vi "MSGR Receive (Name).vi"(0 "MSGR Q name":T2, 11 "error in (no error)":errorcluster, 12 "timeout in ms (-1)":i32=-1) -> (6 "MSGR Q Data TypeDef":T1, 14 "timed out?":bool, 15 "error out":errorcluster)   [LabVIEW 2018]
doc: "$Author::Richard Jennings $\n$Rev:: $\n$Date:: May, 2008 $\n\nOVERVIEW:\nReentrant VI to receive messages via a MSGR Q. If the Q does not exist this VI will create it, then wait for data.\n\nINPUTS (Controls):\n<name> - <short description of each control wired to connector pane>\n\nOUTPUTS (Indicators):\n<name> - <short description of each indicator wired to connector pane>\n\nCopyright 2008 - 2016 Jennings Embedded Servies. All rights reserved.\nAuthor makes no warranties or guarantees related to performance of the software.\nUSE AT YOUR OWN RISK\nwww.jembedded.com"
uses:
  MSGR Q Name TypeDef.ctl
  MSGR Q Data TypeDef.ctl
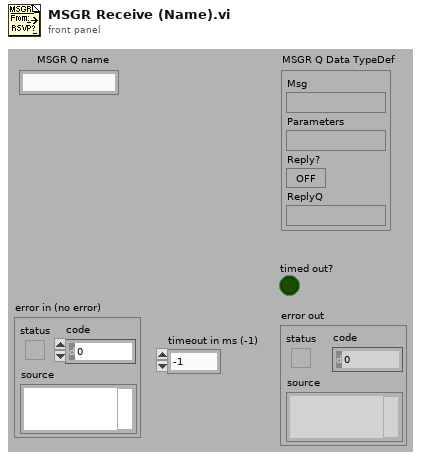
[diagram p1: front panel]
types:
  T1 = typedef "MSGR Q Data TypeDef.ctl" = cluster{"Msg":string, "Parameters":string, "Reply?":bool, "ReplyQ":string}
  T2 = typedef "MSGR Q Name TypeDef.ctl" = string
  T3 = typedef "MSGR Q Ref TypeDef.ctl" = refnum<queue>
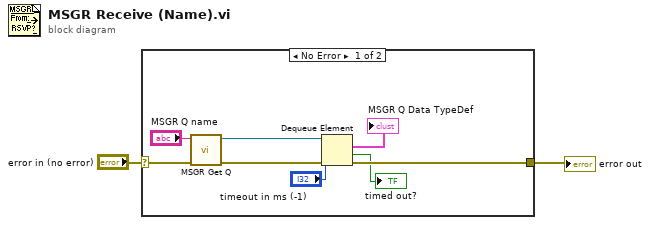
[diagram p0: block diagram]
diagram:
  n1 = case shown="No Error" "error in (no error)" {
    selector: "error in (no error)" -> [w10 w11]
    tunnel: [w6 w11] -> w2
    frame No Error {
      n2 = call "MSGR Get Q.vi"("error in (no error)"=w10, "MSGR Q name"="MSGR Q name") -> ("error out"=w8:errorcluster, "MSGR Q"=w7:T3)  [unwired: 8 out]
      n3 = Dequeue Element(queue=w7, timeout in ms (-1)="timeout in ms (-1)", error in (no error)=w8) -> (element=→"MSGR Q Data TypeDef":T1, timed out?=→"timed out?":bool, error out=w6:errorcluster)  [unwired: 1 out]
    }
    frame Error {
    }
  }
  "error out" <- w2
